vi "Read.vi"(11 "VectoInfoValue in":refnum<class "VectoInfoValue.lvclass">) -> (2 "Vecto Info":T1)   [LabVIEW 2020, in "Vecto.lvlib" / "VectoInfoValue.lvclass"]
uses:
  VectoInfoValue.lvclass
  Connection Type.ctl
  Vecto.lvlib
  Connection Info.ctl
  Vecto Info.ctl
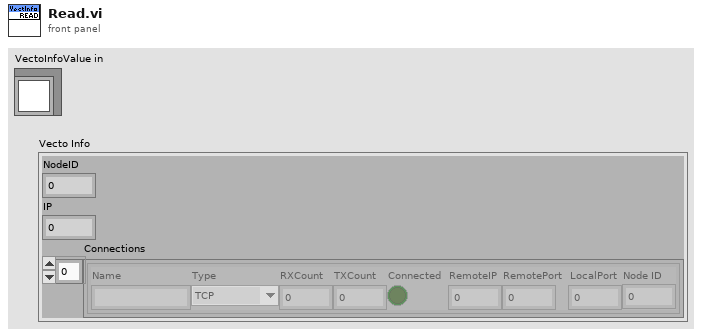
[diagram p1: front panel]
types:
  T1 = typedef "Vecto.lvlib/Vecto Info.ctl" = cluster{"NodeID":i32, "IP":u32, "Connections":T2[]}
  T2 = typedef "Vecto.lvlib/Connection Info.ctl" = cluster{"Name":string, "Type":T3, "RXCount":i32, "TXCount":i32, "Connected":bool, "RemoteIP":u32, "RemotePort":u16, "LocalPort":u16, "Node ID":u32}
  T3 = typedef "Vecto.lvlib/Connection Type.ctl" = enum16{"TCP", "Telemetry", "Discovery", "HTTP"}
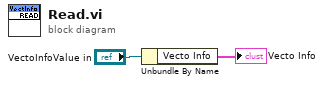
[diagram p0: block diagram]
diagram:
  n1 = Unbundle By Name("VectoInfoValue in") -> ("Vecto Info"=→"Vecto Info":T1)
